vi "Get as Variant.vi"(7 "Variant (Data Type)":variant, 8 "error in (no error)":errorcluster, 10 "Name Array":string[](array[string]), 11 "JSON in":refnum<class "JSON Value.lvclass">) -> (0 "error out":errorcluster, 2 "Variant out":variant, 3 "JSON out":refnum<class "JSON Value.lvclass">)   [LabVIEW 2011, in "Variant JSON.lvlib"]
doc: "Converts a <b>JSON Value</b> into a <b>LabVIEW Variant</b>.\nThe data type of the Variant must be provided. \n\nCopyright 2012 James David Powell, Shaun Rumbell and Ton Plomp\nMore information on http://lavag.org/topic/16217-cr-json-labview"
uses:
  Variant JSON.lvlib
  JSON Value/JSON Value.lvclass
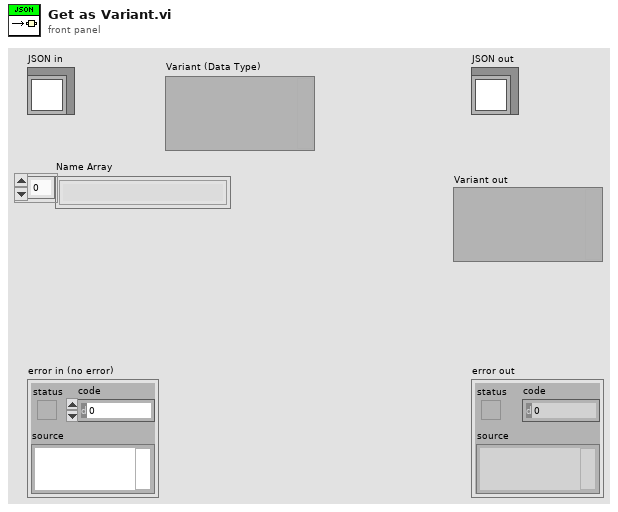
[diagram p1: front panel]
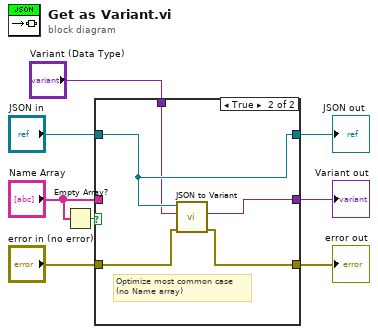
[diagram p0: block diagram]
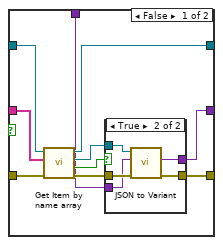
[diagram p2: hidden frame]
diagram:
  n1 = Empty Array?(array="Name Array") -> (empty?=w1:bool)
  n2 = case shown="True" w1 {
    tunnel: "Name Array" -> [w18 _]
    tunnel: "JSON in" -> [w17 w29]
    tunnel: "error in (no error)" -> [w16 w26]
    tunnel: [w12 w25] -> w6
    tunnel: [w11 w29] -> w5
    tunnel: [w10 w28] -> w4
    tunnel: "Variant (Data Type)" -> [w9 w27]
    frame False {
      n3 = call "Get Item by name array.vi"("error in (no error)"=w16, "Name Array"=w18, "JSON Value In"=w17) -> ("error out"=w13:errorcluster, "found"=w14:bool, "Value"=w15:refnum<class "JSON Value.lvclass">, "JSON Value Out"=w11:refnum<class "JSON Value.lvclass">)  [unwired: 5 in]
      n4 = case shown="True" w14 {
        tunnel: w15 -> [_ w24]
        tunnel: w13 -> [w19 w23]
        tunnel: [w19 w22] -> w12
        tunnel: [_ w21] -> w10
        tunnel: w9 -> [_ w20]
        frame False {
        }
        frame True {
          n5 = call "JSON to Variant.vi"("error in (no error)"=w23, "Variant (Data Type)"=w20, "JSON Value"=w24) -> ("error out"=w22:errorcluster, "Variant out"=w21:variant)  [unwired: 7 in]
        }
      }
    }
    frame True {
      # "Optimize most common case\n(no Name array)"
      n6 = call "JSON to Variant.vi"("error in (no error)"=w26, "Variant (Data Type)"=w27, "JSON Value"=w29) -> ("error out"=w25:errorcluster, "Variant out"=w28:variant)  [unwired: 7 in]
    }
  }
  "error out" <- w6
  "JSON out" <- w5
  "Variant out" <- w4
